vi "Edit Config.vi"(8 "error in (no error)":errorcluster, 11 "Polynomial in":refnum<class "Polynomial.lvclass">) -> (0 "error out":errorcluster, 3 "Polynomial out":refnum<class "Polynomial.lvclass">)   [LabVIEW 2024, in "Polynomial.lvclass"]
doc: "Polynomial.lvclass:Edit Config.vi\n\nThis VI is the configuration editor user interface for the Polynomial class.\n\nInstrument Communication Module Version 1.0\nSeptember, 2017 Original Code Consulting David Thomson\n www.originalcode.com"
uses:
  Polynomial.lvclass
  ICM Editor Command.ctl
  ICM Class Editor State.ctl
  ICM Config Command.ctl
  Polynomial.lvclass/Polynomial.ctl
panel:
  in  "New Instance":string
  in  "Delete":bool
  in  "Add":bool
  in  "Revert Scaling":bool
  in  "Instance":u16(ring) items=["1/100th"]
  in  "Save":bool
  out "Order":string[](array[string])=["0th (constant)", "1st (linear)", "2nd (quadratic)", "3rd", "4th", "5th", "6th", "7th", "etc..."]
  in  "Polynomial":dbl[](array[numeric])
  # "To Add New Scaling:\n1. Enter name in New Instance\n2.Click Add New\n3.Select Name in Instance\n4.Adjust Polynomial for desired scaling"
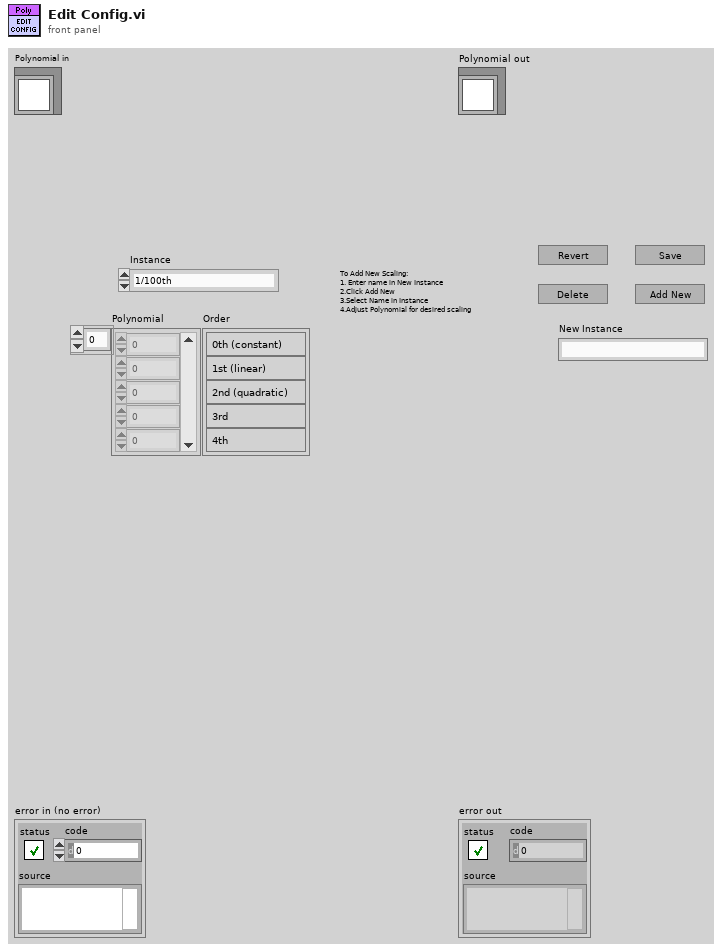
[diagram p1: front panel]
types:
  T1 = typedef "ICM Config Command.ctl" = enum16{"No-op", "Re-Display Sc."}
  T2 = typedef "ICM Class Editor State.ctl" = enum16{"Init", "Wait", "Write", "Read", "Display", "Set Flashing", "Error", "Stop"}
  T3 = typedef "ICM Editor Command.ctl" = enum16{"No-op", "Exit"}
  T4 = enum8{"Enabled", "Disabled", "Disabled and Grayed Out"}
  T5 = cluster{"RingText.Text":string, "Polynomial":dbl[]}
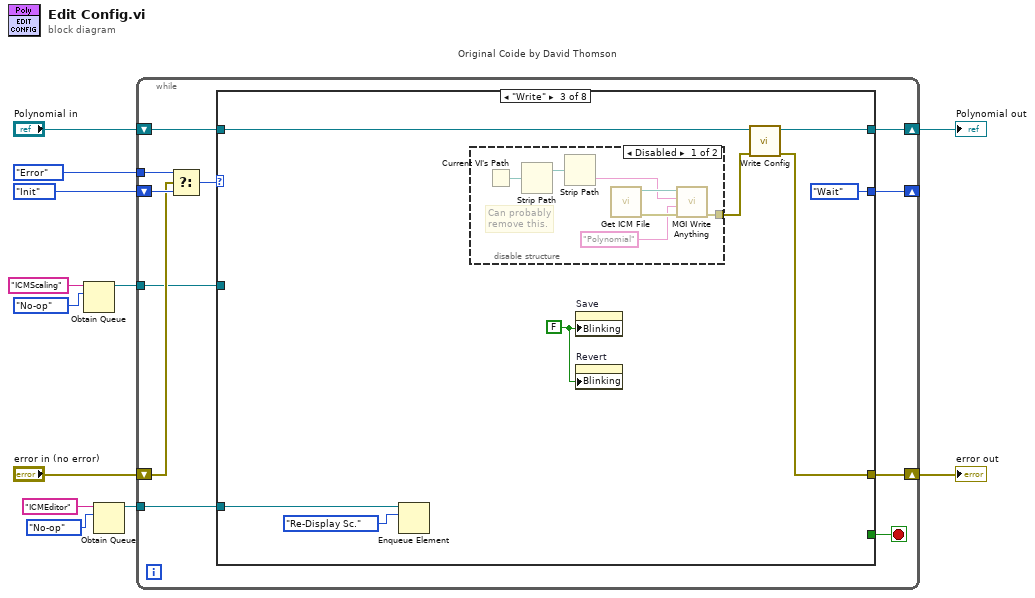
[diagram p0: block diagram]
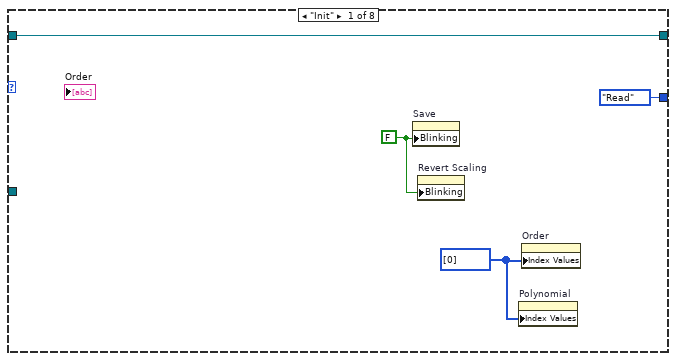
[diagram p2: hidden frame]
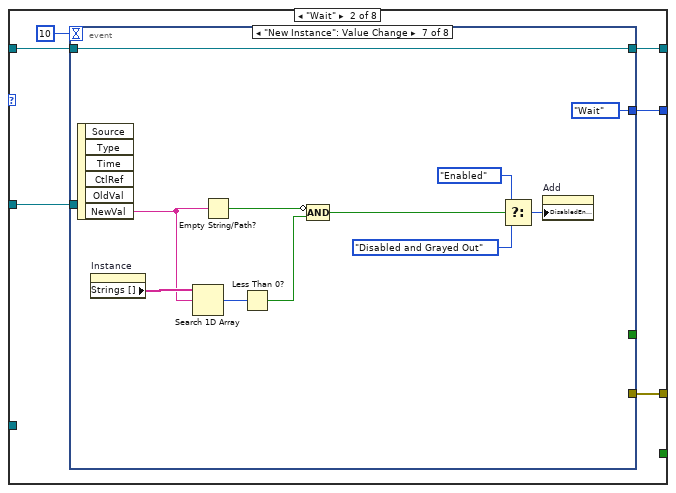
[diagram p3: hidden frame]
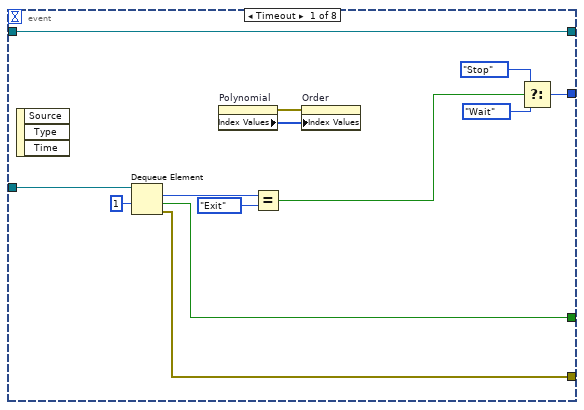
[diagram p4: hidden frame]
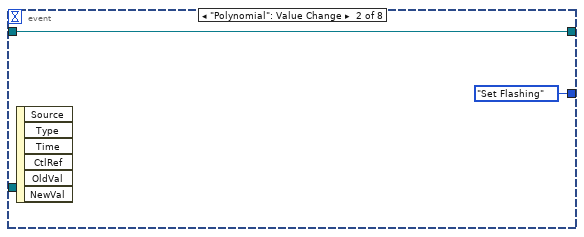
[diagram p5: hidden frame]
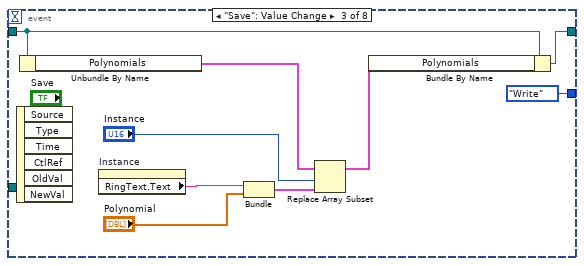
[diagram p6: hidden frame]
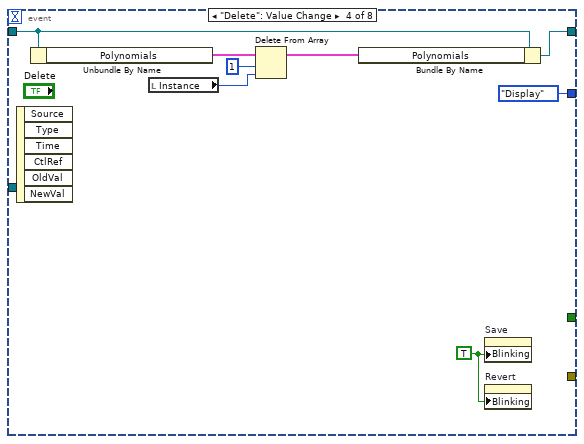
[diagram p7: hidden frame]
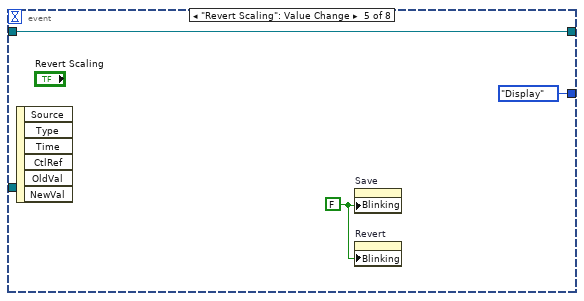
[diagram p8: hidden frame]
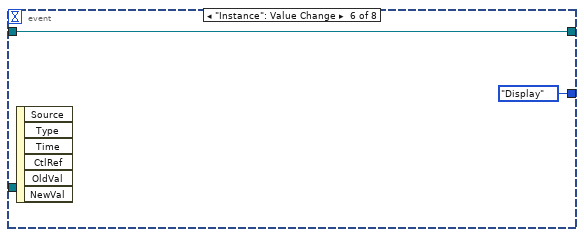
[diagram p9: hidden frame]
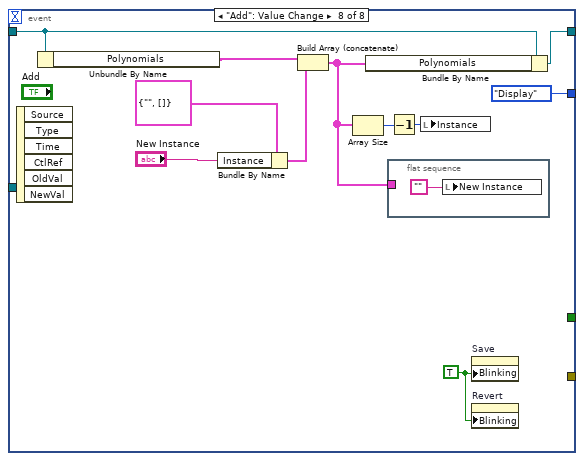
[diagram p10: hidden frame]
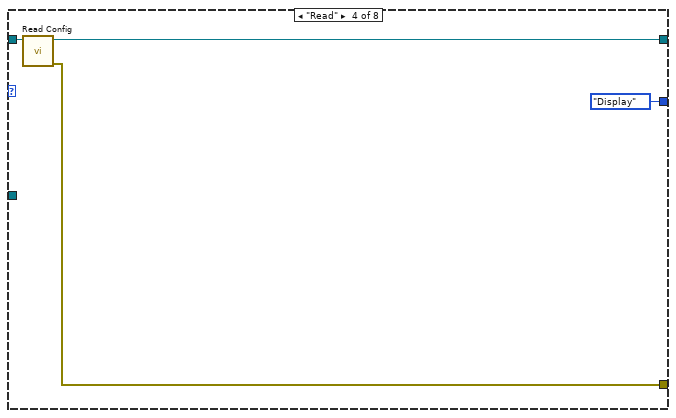
[diagram p12: hidden frame]
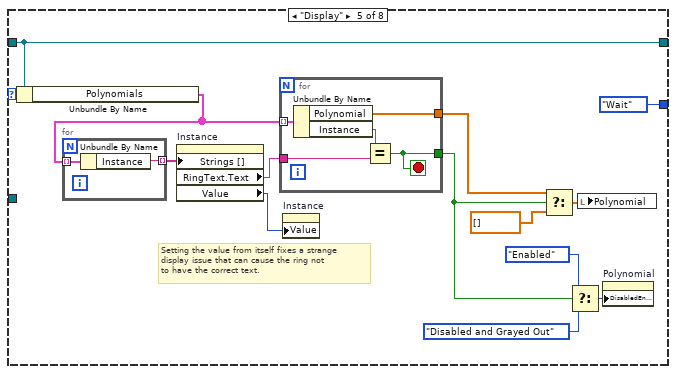
[diagram p13: hidden frame]
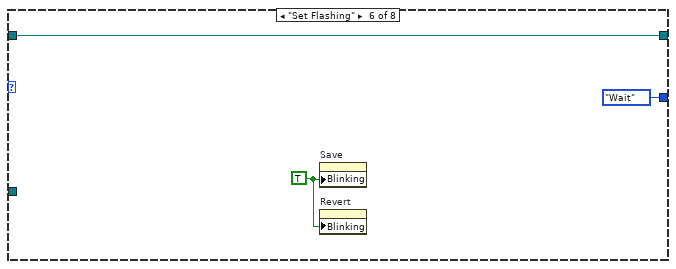
[diagram p14: hidden frame]
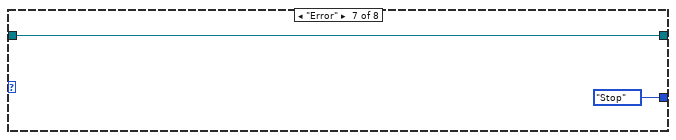
[diagram p15: hidden frame]
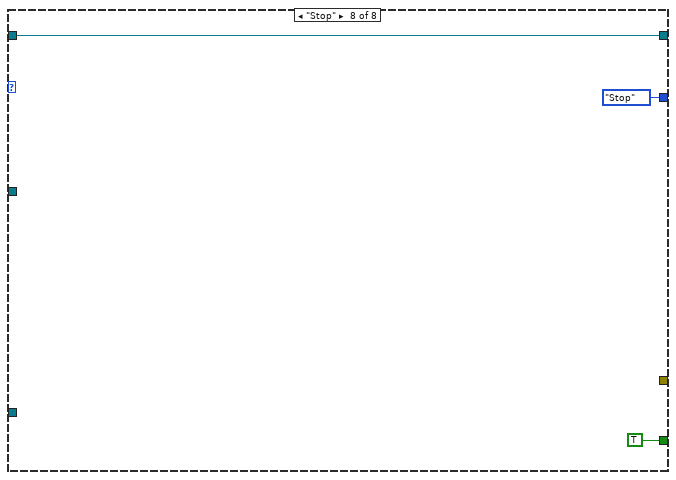
[diagram p16: hidden frame]
diagram:
  n1 = Obtain Queue(name (unnamed)="ICMScaling", element data type=ICM_Editor_Command."No-op" ("Editor Command")) -> (queue out=w8:refnum<queue>)  [unwired: 3 in, 2 out]
  n2 = Obtain Queue(name (unnamed)="ICMEditor", element data type=ICM_Config_Command."No-op" ("Editor Command")) -> (queue out=w1:refnum<queue>)  [unwired: 3 in, 2 out]
  n3 = while "Original Coide by David Thomson" {
    shift-right: [w23] -> w11
    shift-left: "Polynomial in" -> [w22]
    shift-right: [w16] -> _
    shift-left: ICM_Class_Editor_State."Init" ("Config State") -> [w20]
    shift-right: [w15] -> w4
    shift-left: "error in (no error)" -> [w18]
    tunnel: ICM_Class_Editor_State."Error" ("Config State") -> [w17]
    tunnel: w8 -> [w14]
    tunnel: w1 -> [w13]
    stop <- w21 stop-if-true
    n4 = Select(t=w17, s=w18, f=w20) -> (s? t:f=w19:T2)
    n5 = case shown="\"Write\"" w19 {
      tunnel: [w26 w31 w100 w109 w122 w135 w137 w140] -> w23
      tunnel: w22 -> [w26 w30 w97 w111 w122 w135 w137 w140]
      tunnel: [_ _ _ _ _ _ _ TRUE] -> w21
      tunnel: [ICM_Class_Editor_State."Read" ("Config State") w32 ICM_Class_Editor_State."Wait" ("Config State") ICM_Class_Editor_State."Display" ("Config State") ICM_Class_Editor_State."Wait" ("Config State") ICM_Class_Editor_State."Wait" ("Config State") ICM_Class_Editor_State."Stop" ("Config State") ICM_Class_Editor_State."Stop" ("Config State")] -> w16
      tunnel: [_ w28 w99 w110 _ _ _ _] -> w15
      tunnel: w14 -> [_ w29 _ _ _ _ _ _]
      tunnel: w13 -> [_ _ w95 _ _ _ _ _]
      frame "Init" {
        w24 = FALSE ("Blinking")
        w25 = u32[] [0] ("Index Values")
        n6 = property on="Save" class="Bool"("Blinking"=w24) -> ()  [unwired: 2 in, 2 out]
        n7 = property on="Revert Scaling" class="Bool"("Blinking"=w24) -> ()  [unwired: 2 in, 2 out]
        n8 = property on="Polynomial" class="Arr (strict)"("Index Values"=w25) -> ()  [unwired: 2 in, 2 out]
        n9 = property on="Order" class="Arr (strict)"("Index Values"=w25) -> ()  [unwired: 2 in, 2 out]
      }
      frame "Wait" {
        n10 = event shown="[6] \"New Instance\": Value Change" {
          selector: _ -> [_ _ _ _ _ _ _ _]
          dyn-events: _ -> [_ _ _ _ _ _ _ _]
          timeout: 10 -> [_ _ _ _ _ _ _ _]
          tunnel: [w43 ICM_Class_Editor_State."Set Flashing" ("Config State") ICM_Class_Editor_State."Write" ("Config State") ICM_Class_Editor_State."Display" ("Config State") ICM_Class_Editor_State."Display" ("Config State") ICM_Class_Editor_State."Display" ("Config State") ICM_Class_Editor_State."Wait" ("Config State") ICM_Class_Editor_State."Display" ("Config State")] -> w32
          tunnel: [w46 w48 w56 w58 w68 w70 w81 w90] -> w31
          tunnel: w30 -> [w46 w48 w55 w60 w68 w70 w81 w89]
          tunnel: w29 -> [w45 _ _ _ _ _ _ _]
          tunnel: [w37 _ _ _ _ _ _ _] -> w28
          tunnel: [w36 _ _ _ _ _ _ _] -> _
          event Timeout {
            n11 = event-data() -> ()  [unwired: 1 in, 3 out]
            n12 = Dequeue Element(queue=w45, timeout in ms (-1)=1) -> (element=w42:T3, timed out?=w36:bool, error out=w37:errorcluster)  [unwired: 1 in, 1 out]
            n13 = property on="Polynomial" class="Arr (strict)"() -> (error out=w35:errorcluster, "Index Values"=w34:u32[])  [unwired: 2 in, 1 out]
            n14 = Equal?(x=w42, y=ICM_Editor_Command."Exit") -> (x = y?=w40:bool)
            n15 = property on="Order" class="Arr (strict)"(error in=w35, "Index Values"=w34) -> ()  [unwired: 1 in, 2 out]
            n16 = Select(t=ICM_Class_Editor_State."Stop" ("Config State"), s=w40, f=ICM_Class_Editor_State."Wait" ("Config State")) -> (s? t:f=w43:T2)
          }
          event "Polynomial": Value Change {
            n17 = event-data() -> ()  [unwired: 1 in, 6 out]
          }
          event "Save": Value Change {
            n18 = event-data() -> ()  [unwired: 1 in, 6 out]
            n19 = Unbundle By Name(w55) -> ("Polynomials"=w52:cluster{"Instance":string, "Polynomial":dbl[]}[])
            n20 = property on="Instance" class="Ring (strict)"() -> ("RingText.Text"=w50:string)  [unwired: 2 in, 2 out]
            n21 = Bundle("RingText.Text"=w50, "Polynomial"="Polynomial") -> (w53:T5)  [unwired: 1 in]
            n22 = Replace Array Subset(array=w52, new element=w53, index="Instance") -> (w51:cluster{"Instance":string, "Polynomial":dbl[]}[])
            n23 = Bundle By Name(cluster=w55, "Polynomials"=w51) -> (w56:refnum<class "Polynomial.lvclass">)
          }
          event "Delete": Value Change {
            w64 = TRUE ("Blinking")
            n24 = event-data() -> ()  [unwired: 1 in, 6 out]
            n25 = Unbundle By Name(w60) -> ("Polynomials"=w63:cluster{"Instance":string, "Polynomial":dbl[]}[])
            n26 = local read "Instance"() -> (w62:u16)
            n27 = Delete From Array(array=w63, length=1, index=w62) -> (array with subset deleted=w59:cluster{"Instance":string, "Polynomial":dbl[]}[])  [unwired: 1 out]
            n28 = Bundle By Name(cluster=w60, "Polynomials"=w59) -> (w58:refnum<class "Polynomial.lvclass">)
            n29 = property on="Save" class="Bool"("Blinking"=w64) -> ()  [unwired: 2 in, 2 out]
            n30 = property on="Revert" class="Bool"("Blinking"=w64) -> ()  [unwired: 2 in, 2 out]
          }
          event "Revert Scaling": Value Change {
            w66 = FALSE ("Blinking")
            n31 = event-data() -> ()  [unwired: 1 in, 6 out]
            n32 = property on="Save" class="Bool"("Blinking"=w66) -> ()  [unwired: 2 in, 2 out]
            n33 = property on="Revert" class="Bool"("Blinking"=w66) -> ()  [unwired: 2 in, 2 out]
          }
          event "Instance": Value Change {
            n34 = event-data() -> ()  [unwired: 1 in, 6 out]
          }
          event "New Instance": Value Change {
            n35 = event-data() -> ("NewVal"=w73:string)  [unwired: 1 in, 5 out]
            n36 = property on="Instance" class="Ring (strict)"() -> ("Strings []"=w74:string[])  [unwired: 2 in, 2 out]
            n37 = Search 1D Array(1D array=w74, element=w73) -> (index of element=w72:i32)  [unwired: 1 in]
            n38 = Empty String/Path?(string/path=w73) -> (empty?=w76:bool)
            n39 = Less Than 0?(x=w72) -> (x < 0?=w71:bool)
            n40 = Compound Arithmetic op=AND(invert w76, w71) -> (w75:bool)
            n41 = Select(t=T4."Enabled" ("Disabled"), s=w75, f=T4."Disabled and Grayed Out" ("Disabled")) -> (s? t:f=w79:T4)
            n42 = property on="Add" class="Bool"("DisabledEnum"=w79) -> ()  [unwired: 2 in, 2 out]
          }
          event "Add": Value Change {
            w92 = TRUE ("Blinking")
            n43 = event-data() -> ()  [unwired: 1 in, 6 out]
            n44 = Unbundle By Name(w89) -> ("Polynomials"=w88:cluster{"Instance":string, "Polynomial":dbl[]}[])
            n45 = Bundle By Name(cluster=cluster{"Instance":string, "Polynomial":dbl[]} {"Instance"="", "Polynomial"=[]} ("Cluster"), "Instance"="New Instance") -> (w86:cluster{"Instance":string, "Polynomial":dbl[]})
            n46 = Build Array (concatenate)(w88, w86) -> (w82:cluster{"Instance":string, "Polynomial":dbl[]}[])
            n47 = Array Size(array=w82) -> (size(s)=w84:i32)
            n48 = Bundle By Name(cluster=w89, "Polynomials"=w82) -> (w90:refnum<class "Polynomial.lvclass">)
            n49 = flat-sequence {
              tunnel: w82 -> [_]
              frame #0 {
                n50 = local write "New Instance"("") -> ()
              }
            }
            n51 = Decrement(x=w84) -> (x-1=w83:i32)
            n52 = local write "Instance"(w83) -> ()
            n53 = property on="Save" class="Bool"("Blinking"=w92) -> ()  [unwired: 2 in, 2 out]
            n54 = property on="Revert" class="Bool"("Blinking"=w92) -> ()  [unwired: 2 in, 2 out]
          }
        }
      }
      frame "Write" {
        w96 = FALSE ("Blinking")
        n55 = Enqueue Element(queue=w95, element=ICM_Config_Command."Re-Display Sc.") -> ()  [unwired: 2 in, 3 out]
        n56 = disable-structure shown="Disabled" {
          disable-tunnel: [w104 _] -> w98
          frame Disabled {
            # "Can probably\nremove this."
            n57 = Current VI's Path() -> (path=w108:path)
            n58 = Strip Path(path=w108) -> (stripped path=w107:path)  [unwired: 1 out]
            n59 = Strip Path(path=w107) -> (name=w103:string)  [unwired: 1 out]
            n60 = call "Get ICM File.vi"() -> ("error out"=w105:errorcluster, "ICM File"=w106:path)  [unwired: 10 in]
            n61 = call "MGI Write Anything.vi"("Error In"=w105, "Section Name (Name of \"Anything\")"="Polynomial" ("Section Name (Name of \"Anything\")"), "Anything"=w103, "Path (dialog)"=w106) -> ("Error Out"=w104:errorcluster)  [unwired: 5 in, 2 out]
          }
          frame Enabled {
          }
        }
        n62 = property on="Save" class="Bool"("Blinking"=w96) -> ()  [unwired: 2 in, 2 out]
        n63 = property on="Revert" class="Bool"("Blinking"=w96) -> ()  [unwired: 2 in, 2 out]
        n64 = call-dynamic "Write Config.vi"("error in (no error)"=w98, "Polynomial in"=w97) -> ("error out"=w99:errorcluster, "Polynomial out"=w100:refnum<class "Polynomial.lvclass">)  [unwired: 8 in]
      }
      frame "Read" {
        n65 = call-dynamic "Read Config.vi"("Polynomial in"=w111) -> ("error out"=w110:errorcluster, "Polynomial out"=w109:refnum<class "Polynomial.lvclass">)  [unwired: 9 in]
      }
      frame "Display" {
        # "Setting the value from itself fixes a strange\ndisplay issue that can cause the ring not\nto have the correct text."
        n66 = Unbundle By Name(w122) -> ("Polynomials"=w117:cluster{"Instance":string, "Polynomial":dbl[]}[])
        n67 = for {
          tunnel: w117 -> [w132] mode=indexing
          tunnel: [w131] -> w118 mode=indexing
          n68 = Unbundle By Name(w132) -> ("Instance"=w131:string)
        }
        n69 = property on="Instance" class="Ring (strict)"("Strings []"=w118) -> ("RingText.Text"=w116:string, "Value"=w113:u16)  [unwired: 2 in, 2 out]
        n70 = for {
          tunnel: w117 -> [w130] mode=indexing
          tunnel: w116 -> [w128]
          tunnel: [w127] -> w114
          tunnel: [w126] -> w115
          stop <- w127 stop-if-true
          n71 = Unbundle By Name(w130) -> ("Polynomial"=w126:dbl[], "Instance"=w129:string)
          n72 = Equal?(x=w129, y=w128) -> (x = y?=w127:bool)
        }
        n73 = property on="Instance" class="Ring (strict)"("Value"=w113) -> ()  [unwired: 2 in, 2 out]
        n74 = Select(t=w115, s=w114, f=dbl[] []) -> (s? t:f=w124:dbl[])
        n75 = Select(t=T4."Enabled" ("Disabled"), s=w114, f=T4."Disabled and Grayed Out" ("Disabled")) -> (s? t:f=w121:T4)
        n76 = local write "Polynomial"(w124) -> ()
        n77 = property on="Polynomial" class="Arr (strict)"("DisabledEnum"=w121) -> ()  [unwired: 2 in, 2 out]
      }
      frame "Set Flashing" {
        w133 = TRUE ("Blinking")
        n78 = property on="Save" class="Bool"("Blinking"=w133) -> ()  [unwired: 2 in, 2 out]
        n79 = property on="Revert" class="Bool"("Blinking"=w133) -> ()  [unwired: 2 in, 2 out]
      }
      frame "Error" {
      }
      frame "Stop" {
      }
    }
  }
  "error out" <- w4
  "Polynomial out" <- w11
